vi "ge_SimMouse.vi"(7 "error in":errorcluster, 8 "CtrlPos":T1) -> (0 "error out":errorcluster)   [LabVIEW 2012]
uses:
  <vilib>/Utility/miscctls.llb/LVPositionTypeDef.ctl
  user32.dll
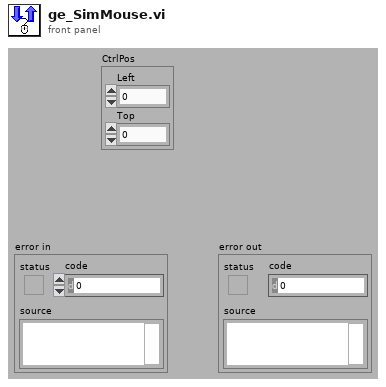
[diagram p1: front panel]
types:
  T1 = typedef "LVPositionTypeDef.ctl" = cluster{"Left":i32, "Top":i32}
  T2 = typedef "LVRectTypeDef.ctl" = cluster{"left":i16, "top":i16, "right":i16, "bottom":i16}
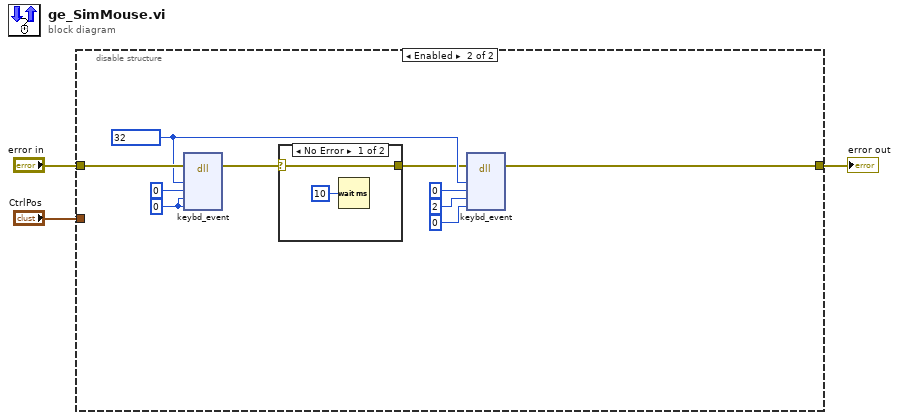
[diagram p0: block diagram]
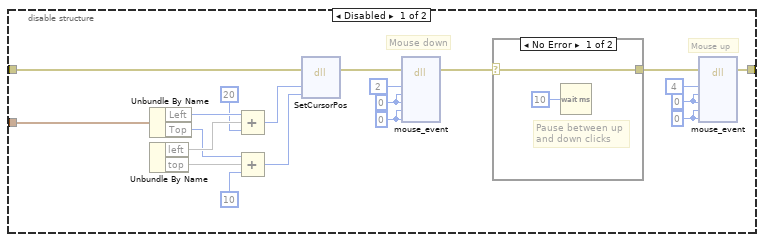
[diagram p2: hidden frame]
diagram:
  n1 = disable-structure shown="Enabled" {
    disable-tunnel: [w24 w30] -> w3
    disable-tunnel: "CtrlPos" -> [w14 _]
    disable-tunnel: "error in" -> [w4 w37]
    frame Disabled {
      w18 = u32 0 ("dwExtraInfo")
      w20 = 0 ("dx")
      w21 = u32 0 ("dwExtraInfo")
      w23 = 0 ("dx")
      # "Mouse up"
      # "Mouse down"
      n2 = Unbundle By Name(w14) -> ("Left"=w13:i32, "Top"=w10:i32)
      n3 = Unbundle By Name() -> (w6:T2, "left"=w12, "top"=w11)
      n4 = Compound Arithmetic op=ADD(w13, w12, i16 20 ("value")) -> (w8:i32)
      n5 = Compound Arithmetic op=ADD(w10, w11, i16 10 ("value")) -> (w7:i32)
      n6 = dll-call lib="user32.dll" fn="SetCursorPos"(error in=w4, "dx"=w8, "dy"=w7) -> (error out=w15:errorcluster)  [unwired: 5 in, 1 out]
      n7 = dll-call lib="User32.dll" fn="mouse_event"(error in=w15, "dwFlags"=u32 2, "dx"=w23, "dy"=w23, "dwData"=w21, "dwExtraInfo"=w21) -> (error out=w17:errorcluster)  [unwired: 7 in, 2 out]
      n8 = case shown="No Error" w17 {
        selector: w17 -> [w25 w27]
        tunnel: [w25 w27] -> w16
        frame No Error {
          # "Pause between up \nand down clicks"
          n9 = Wait (ms)(milliseconds to wait=u32 10) -> ()  [unwired: 1 out]
        }
        frame Error {
        }
      }
      n10 = dll-call lib="User32.dll" fn="mouse_event"(error in=w16, "dwFlags"=u32 4, "dx"=w20, "dy"=w20, "dwData"=w18, "dwExtraInfo"=w18) -> (error out=w24:errorcluster)  [unwired: 7 in, 2 out]
    }
    frame Enabled {
      w35 = u32 0 ("dwExtraInfo")
      w32 = u8 32 ("Virtual Key")
      n11 = dll-call lib="user32.dll" fn="keybd_event"(error in=w37, "bVk"=w32, "bScan"=u8 0, "dwFlags"=w35, "dwExtraInfo"=w35) -> (error out=w29:errorcluster)  [unwired: 7 in, 1 out]
      n12 = case shown="No Error" w29 {
        selector: w29 -> [w39 w40]
        tunnel: [w39 w40] -> w28
        frame No Error {
          n13 = Wait (ms)(milliseconds to wait=u32 10) -> ()  [unwired: 1 out]
        }
        frame Error {
        }
      }
      n14 = dll-call lib="user32.dll" fn="keybd_event"(error in=w28, "bVk"=w32, "bScan"=u8 0, "dwFlags"=u32 2, "dwExtraInfo"=u32 0) -> (error out=w30:errorcluster)  [unwired: 7 in, 1 out]
    }
  }
  "error out" <- w3
